vi "2.34.vi"(1 "数值 3":dbl, 2 "数值 2":dbl, 3 "数值":dbl) -> (0 "数值 4":dbl)   [LabVIEW 2017]
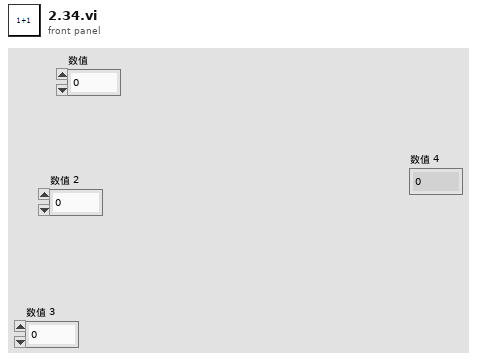
[diagram p1: front panel]
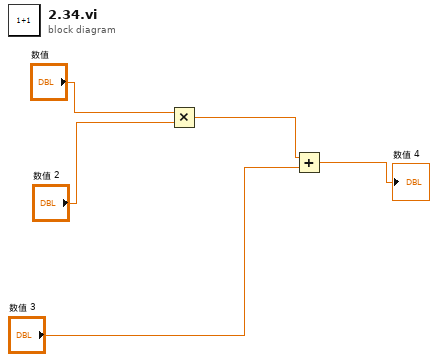
[diagram p0: block diagram]
diagram:
  n1 = Multiply(x="数值", y="数值 2") -> (x*y=w2:dbl)
  n2 = Add(x=w2, y="数值 3") -> (x+y=→"数值 4":dbl)
